vi "Shorting of Test Seq Program.vi"(5 "Feature List (Out)":T1(array[cluster])) -> (1 "Feature Step Enable":T1(array[cluster]), 2 "Feature Name":string[][](array[string]))   [LabVIEW 2015]
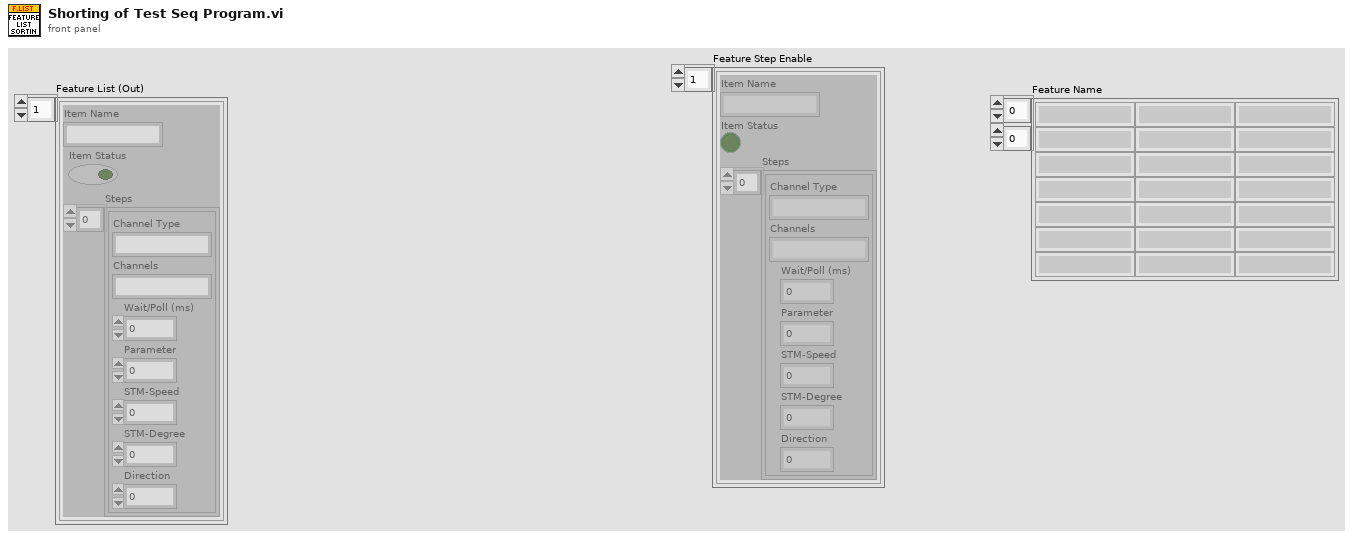
[diagram p1: front panel]
types:
  T1 = cluster{"Item Name":string, "Item Status":bool, "Steps":cluster{"Channel Type":string, "Channels":string, "Wait/Poll (ms)":u32, "Parameter":u8, "STM-Speed":i32, "STM-Degree":u32, "Direction":u8}[]}[]
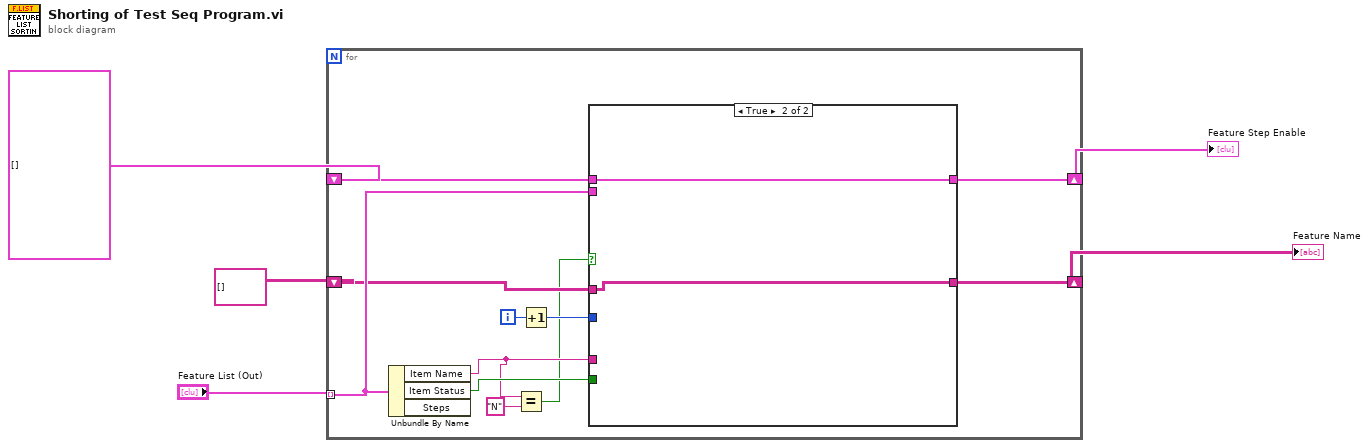
[diagram p0: block diagram]
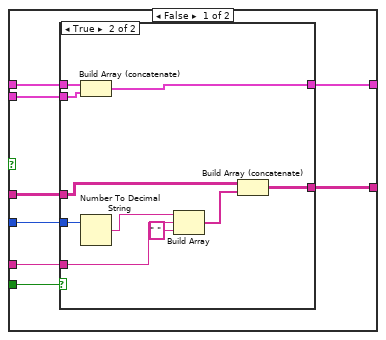
[diagram p2: hidden frame]
diagram:
  n1 = for {
    tunnel: "Feature List (Out)" -> [w15] mode=indexing
    shift-right: [w9] -> w1
    shift-left: string[][] [] -> [w12]
    shift-right: [w11] -> w3
    shift-left: T1 [] -> [w10]
    i -> [w14]
    n2 = Unbundle By Name(w15) -> ("Item Name"=w8:string, "Item Status"=w16:bool)  [unwired: 1 out]
    n3 = Equal?(x=w8, y="N") -> (x = y?=w6:bool)
    n4 = Increment(x=w14) -> (x+1=w13:i32)
    n5 = case shown="True" w6 {
      tunnel: w16 -> [w24 _]
      tunnel: w15 -> [w23 _]
      tunnel: w13 -> [w22 _]
      tunnel: w12 -> [w21 w37]
      tunnel: [w20 w38] -> w11
      tunnel: w10 -> [w19 w38]
      tunnel: [w18 w37] -> w9
      tunnel: w8 -> [w17 _]
      frame False {
        n6 = case shown="True" w24 {
          tunnel: w17 -> [_ w31]
          tunnel: w23 -> [_ w34]
          tunnel: w22 -> [_ w36]
          tunnel: [w25 w28] -> w18
          tunnel: w21 -> [w25 w29]
          tunnel: [w26 w33] -> w20
          tunnel: w19 -> [w26 w32]
          frame False {
          }
          frame True {
            n7 = Build Array (concatenate)(w32, w34) -> (w33:T1)
            n8 = Number To Decimal String(number=w36) -> (decimal integer string=w35:string)  [unwired: 1 in]
            n9 = Build Array(w35, w31, " " ("element")) -> (w27:string[])
            n10 = Build Array (concatenate)(w29, w27) -> (w28:string[][])
          }
        }
      }
      frame True {
      }
    }
  }
  "Feature Name" <- w1
  "Feature Step Enable" <- w3
